vi "Teleop.vi"() -> ()   [LabVIEW 2014]
doc: "This VI is called for each TeleOp packet received from the DS where the robot is not disabled. It is often used to read from the joysticks and update I/O or to update setpoints for timed control loops. It should complete and return within 20 milliseconds or it may miss DS packets."
uses:
  <vilib>/Rock Robotics/WPI/DriverStation/WPI_DriverStationDerivedRobotMode.ctl
  <vilib>/Rock Robotics/WPI/DriverStation/WPI_DriverStationMatch Info.ctl
  <vilib>/Rock Robotics/Network Tables/SD Read Boolean.vi
  <vilib>/Rock Robotics/Network Tables/SD Read Number.vi
  <vilib>/Rock Robotics/WPI/Joystick/WPI_JoystickGetSetRefNum.vi
  <vilib>/Rock Robotics/Network Tables/SD Write Boolean Array.vi
  <vilib>/Rock Robotics/Network Tables/SD Write Numeric Array.vi
  <vilib>/Rock Robotics/Network Tables/SD Write Boolean.vi
  Global 1.vi
  <vilib>/Rock Robotics/WPI/RobotDrive/WPI_RobotDriveGetSetRefNum.vi
panel:
  out "Sample Slider 0":dbl(slide) scale=0.0..5.0
  out "Sample Boolean 1":bool
  out "Sample Boolean 0":bool
  in  "Match Info":T1={"Autonomous Elapsed Seconds"=0.0, "TeleOp Elapsed Seconds"=0.0, "Disabled Elapsed Seconds"=0.0, "Visited Autonomous"=FALSE, "Visited TeleOp"=FALSE, "Visited Disabled"=FALSE, "Autonomous Settings"={"Autonomous Style"=enum."Independent", "VI Refnum"=refnum}}
  in  "Call Context":T2
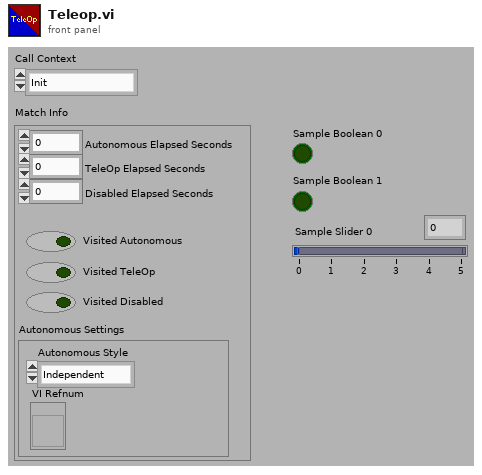
[diagram p1: front panel]
types:
  T1 = typedef "WPI_DriverStationMatch Info.ctl" = cluster{"Autonomous Elapsed Seconds":dbl, "TeleOp Elapsed Seconds":dbl, "Disabled Elapsed Seconds":dbl, "Visited Autonomous":bool, "Visited TeleOp":bool, "Visited Disabled":bool, "Autonomous Settings":cluster{"Autonomous Style":enum16{"Iterative", "Independent"}, "VI Refnum":refnum<vi>}}
  T2 = typedef "WPI_DriverStationDerivedRobotMode.ctl" = enum16{"Init", "Execute", "Stop"}
  T3 = typedef "WPI_RobotDriveDevRef.ctl" = cluster{"DevStatus":errorcluster, "Motors[]":T4[], "Square Inputs":bool, "Max Output":dbl}
  T4 = typedef "WPI_MotorControlDeviceRef.ctl" = cluster{"DeviceStatus":errorcluster, "Type":enum16{"PWM", "CAN"}, "PWM":cluster{"Digital Module":T5, "PWM Channel":T6, "DeadBand":T7}, "CAN":cluster{"Device Number":u8, "Control Mode":T8, "Semaphore":T9, "Max Vout":dbl}, "Invert":bool, "TransformRef":T10, "InvTransformRef":T10}
  T5 = typedef "FPGA_TypedefDigitalModule.ctl" = enum16{"Digital Module 1", "Digital Module 2"}
  T6 = typedef "FPGA_DIOPWMChannel.ctl" = enum8{"PWM 1", "PWM 2", "PWM 3", "PWM 4", "PWM 5", "PWM 6", "PWM 7", "PWM 8", "PWM 9", "PWM 10", "Invalid"}
  T7 = typedef "WPI_PWMDeadband.ctl" = cluster{"Name":string, "maxPositivePwm":i32, "minPositivePwm":i32, "centerPwm":i32, "maxNegativePwm":i32, "minNegativePwm":i32, "angularRange":u16}
  T8 = typedef "WPI_CANJaguar_ControlMode.ctl" = enum8{"Percent VBus", "Current", "Speed", "Position", "Voltage"}
  T9 = typedef "Semaphore RefNum" = refnum<k1>
  T10 = typedef "WPI_PWMTransform_ConPane.ctl" = refnum<vi>
  T11 = typedef "WPI_JoystickDevRef.ctl" = cluster{"Device":T12}
  T12 = typedef "WPI_JoystickDeviceEnum.ctl" = enum16{"USB 0", "USB 1", "USB 2", "USB 3", "USB 4", "USB 5"}
  T13 = typedef "WPI_DigitalInputDevRef.ctl" = cluster{"DevStatus":errorcluster, "DIO Channel":T14, "Digital Module":T5}
  T14 = typedef "FPGA_DIOChannel.ctl" = enum8{"DIO 1", "DIO 2", "DIO 3", "DIO 4", "DIO 5", "DIO 6", "DIO 7", "DIO 8", "DIO 9", "DIO 10", "DIO 11", "DIO 12", "DIO 13", "DIO 14", "Invalid"}
  T15 = typedef "WPI_EncoderDevRef.ctl" = cluster{"DevStatus":errorcluster, "EncoderIndex":T16, "CounterIndex":T17, "DistancePerCount":dbl, "Decoding Type":T18}
  T16 = typedef "FPGA_EncoderIdx.ctl" = enum8{"Enc 0", "Enc 1", "Enc 2", "Enc 3", "Invalid"}
  T17 = typedef "FPGA_CounterCtrSystemIndex.ctl" = enum8{"Ctr 0", "Ctr 1", "Ctr 2", "Ctr 3", "Ctr 4", "Ctr 5", "Ctr 6", "Ctr 7", "Invalid"}
  T18 = typedef "WPI_EncoderType.ctl" = enum16{"1x", "2x", "4x"}
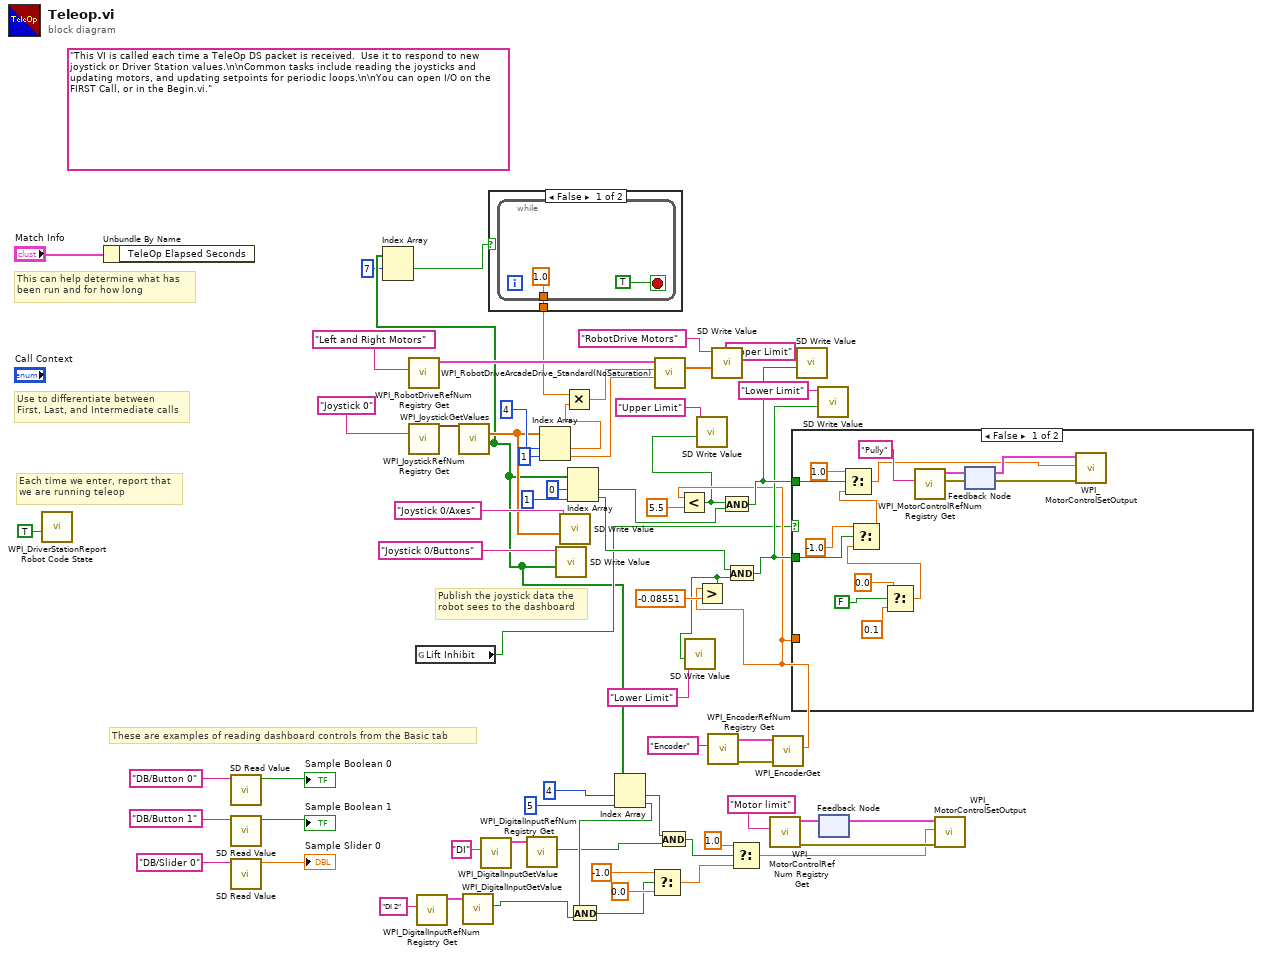
[diagram p0: block diagram]
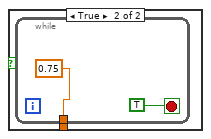
[diagram p2: hidden frame]
diagram:
  (unwired) "This VI is called each time a TeleOp DS packet is received.  Use it to respond to new joystick or Driver Station values.\n\nCommon tasks include reading the joysticks and updating motors, and updating setpoints for periodic loops.\n\nYou can open I/O on the FIRST Call, or in the Begin.vi."
  # "Publish the joystick data the\nrobot sees to the dashboard"
  # "These are examples of reading dashboard controls from the Basic tab"
  # "Each time we enter, report that\nwe are running teleop"
  # "Use to differentiate between\nFirst, Last, and Intermediate calls"
  # "This can help determine what has\nbeen run and for how long"
  n1 = call <vilib>:"WPI_DriverStationReport Robot Code State.vi"("TeleOp"=TRUE ("Autonomous")) -> ()  [unwired: 10 in, 1 out]
  n2 = Unbundle By Name("Match Info") -> ()  [unwired: 1 out]
  n3 = call-poly <vilib>:"SD Read Value.vi"("Name"="DB/Button 0" ("refnum name")) -> ("Boolean"=→"Sample Boolean 0":bool)  [unwired: 8 in, 2 out]
  n4 = call-poly <vilib>:"SD Read Value.vi"("Name"="DB/Button 1" ("refnum name")) -> ("Boolean"=→"Sample Boolean 1":bool)  [unwired: 8 in, 2 out]
  n5 = call-poly <vilib>:"SD Read Value.vi"("Name"="DB/Slider 0" ("refnum name")) -> ("Numeric"=→"Sample Slider 0":dbl)  [unwired: 8 in, 2 out]
  n6 = call <vilib>:"WPI_RobotDriveRefNum Registry Get.vi"("refnum name"="Left and Right Motors") -> ("RobotDriveDevRef"=w22:T3)  [unwired: 1 in, 9 out]
  n7 = call <vilib>:"WPI_JoystickRefNum Registry Get.vi"("refnum name"="Joystick 0") -> ("JoystickDevRef"=w56:T11)  [unwired: 1 in, 9 out]
  n8 = global read "Global 1.vi" "Lift Inhibit"() -> (w5:bool)
  n9 = call <vilib>:"WPI_DigitalInputRefNum Registry Get.vi"("refnum name"="DI 2") -> ("DigitalInputDevRef"=w32:T13)  [unwired: 9 in, 1 out]
  n10 = call <vilib>:"WPI_JoystickGetValues.vi"("JoystickDevRef"=w56) -> ("Buttons"=w3:bool[], "Axes"=w46:dbl[])  [unwired: 6 in, 3 out]
  n11 = Index Array(array=w3, index #1=7 ("index")) -> (element #1=w2:bool)  [unwired: 1 in, 1 out]
  n12 = call <vilib>:"WPI_DigitalInputGetValue.vi"("DigitalInputDevRef"=w32) -> ("Value"=w25:bool)  [unwired: 8 in, 2 out]
  n13 = call <vilib>:"WPI_DigitalInputRefNum Registry Get.vi"("refnum name"="DI") -> ("DigitalInputDevRef"=w34:T13)  [unwired: 9 in, 1 out]
  n14 = case shown="False" w2 {
    tunnel: [w67 w70] -> w4
    frame False {
      n15 = while {
        tunnel: [1.0 ("x")] -> w67
        stop <- TRUE stop-if-true
      }
    }
    frame True {
      n16 = while {
        tunnel: [0.75 ("x")] -> w70
        stop <- TRUE stop-if-true
      }
    }
  }
  n17 = call <vilib>:"WPI_DigitalInputGetValue.vi"("DigitalInputDevRef"=w34) -> ("Value"=w26:bool)  [unwired: 8 in, 2 out]
  n18 = Index Array(array=w46, index #1=4 ("index"), index #2=1 ("index")) -> (element #1=w24:dbl, element #2=w54:dbl)
  n19 = call-poly <vilib>:"SD Write Value.vi"("Boolean Array"=w3, "Name"="Joystick 0/Buttons") -> ()  [unwired: 8 in, 2 out]
  n20 = call-poly <vilib>:"SD Write Value.vi"("Numeric Array"=w46, "Name"="Joystick 0/Axes") -> ()  [unwired: 8 in, 2 out]
  n21 = Multiply(x=w4, y=w24) -> (x*y=w23:dbl)
  n22 = Index Array(array=w3, index #1=0 ("index"), index #2=1 ("index")) -> (element #1=w15:bool, element #2=w17:bool)
  n23 = Index Array(array=w3, index #1=4 ("index"), index #2=5 ("index")) -> (element #1=w30:bool, element #2=w28:bool)
  n24 = And(x=w28, y=w25) -> (x .and. y?=w27:bool)
  n25 = Select(t=-1.0, s=w27, f=0.0) -> (s? t:f=w43:dbl)
  n26 = call <vilib>:"WPI_RobotDriveArcadeDrive_Standard(NoSaturation).vi"("Y axis value"=w54, "X axis value"=w23, "RobotDriveDevRef"=w22) -> ("Motor Values"=w53:dbl[])  [unwired: 1 in, 7 out]
  n27 = And(x=w30, y=w26) -> (x .and. y?=w29:bool)
  n28 = call <vilib>:"WPI_EncoderRefNum Registry Get.vi"("refnum name"="Encoder") -> ("error out"=w21:errorcluster, "EncoderDevRef"=w20:T15)  [unwired: 9 in]
  n29 = call-poly <vilib>:"SD Write Value.vi"("Numeric Array"=w53, "Name"="RobotDrive Motors") -> ()  [unwired: 8 in, 2 out]
  n30 = Select(t=1.0, s=w29, f=w43) -> (s? t:f=w35:dbl)
  n31 = call <vilib>:"WPI_EncoderGet.vi"("error in (no error)"=w21, "EncoderDevRef"=w20) -> ("Distance"=w10:dbl)  [unwired: 4 in, 5 out]
  n32 = Less?(x=w10, y=5.5) -> (x < y?=w7:bool)
  n33 = call-poly <vilib>:"SD Write Value.vi"("Boolean"=w7, "Name"="Upper Limit") -> ()  [unwired: 8 in, 2 out]
  n34 = Greater?(x=w10, y=-0.08551) -> (0:w9:bool)
  n35 = call-poly <vilib>:"SD Write Value.vi"("Boolean"=w9, "Name"="Lower Limit") -> ()  [unwired: 8 in, 2 out]
  n36 = And(x=w7, y=w15) -> (x .and. y?=w14:bool)
  n37 = And(x=w17, y=w9) -> (x .and. y?=w13:bool)
  n38 = case shown="False" w5 {
    tunnel: w14 -> [w86 _]
    tunnel: w13 -> [w84 _]
    tunnel: w10 -> [_ _]
    frame False {
      n39 = Select(t=0.0, s=FALSE, f=0.1) -> (s? t:f=w76:dbl)
      n40 = Select(t=-1.0, s=w84, f=w76) -> (s? t:f=w82:dbl)
      n41 = Select(t=1.0, s=w86, f=w82) -> (s? t:f=w77:dbl)
      n42 = feedback #1() -> (w78:T4)  [unwired: 1 in]
      n43 = call <vilib>:"WPI_MotorControlSetOutput.vi"("Output"=w77, "MotorControlDevRef"=w78) -> ("error out"=w81:errorcluster)  [unwired: 7 in, 2 out]
      n44 = call <vilib>:"WPI_MotorControlRefNum Registry Get.vi"("error in (no error)"=w81, "refnum name"="Pully") -> ("MotorControlDevRef"=w79:T4)  [unwired: 8 in, 1 out]
      n45 = feedback-in #1(w79) -> ()
    }
    frame True {
    }
  }
  n46 = call-poly <vilib>:"SD Write Value.vi"("Boolean"=w14, "Name"="Upper Limit") -> ()  [unwired: 8 in, 2 out]
  n47 = call-poly <vilib>:"SD Write Value.vi"("Boolean"=w13, "Name"="Lower Limit") -> ()  [unwired: 8 in, 2 out]
  n48 = feedback #2() -> (w36:T4)  [unwired: 1 in]
  n49 = call <vilib>:"WPI_MotorControlSetOutput.vi"("Output"=w35, "MotorControlDevRef"=w36) -> ("error out"=w39:errorcluster)  [unwired: 7 in, 2 out]
  n50 = call <vilib>:"WPI_MotorControlRefNum Registry Get.vi"("error in (no error)"=w39, "refnum name"="Motor limit") -> ("MotorControlDevRef"=w37:T4)  [unwired: 8 in, 1 out]
  n51 = feedback-in #2(w37) -> ()
